vi "svc_ Octave Spectrum Labels and Units.vi"(9 "octave info":T1={"standard"=enum."ANSI S1.11", "bandwidth"=enum."1 octave", "low band"=0, "high band"=0, "weighting filter"=0, "dB reference"=0.0, "dB On"=FALSE, "unit label"="", "channel name"="", "description"="", "engineering units"=1, "custom label"="", "spectrum type"=enum."magnitude", "spectral density"=FALSE, "filters settled"=FALSE} {"engineering units" items=["custom..."=0, "V"=1, "A"=21, "C"=30, "pC"=31, "s"=32, "-"=29, "Pa"=2, "N"=20, "g"=3, "m/s^2"=4, "m/s"=5, "m"=6, "mm/s"=12, "mm"=13, "micron/s"=14, "micron"=15, "in/s^2"=7, "in/s"=8, "in"=9, "mil/s"=10, "mil"=11, "rad/s^2"=16, "rad/s"=17, "rad"=18, "deg/s^2"=26, "deg/s"=27, "deg"=28, "RPM"=22, "cycle/s^2"=23, "Hz"=24, "cycle"=25, "strain"=19]; "dB reference" format="%.2e"; "weighting filter" items=["Linear", "A-weighting", "B-weighting", "C-weighting", "ITU-R 468-4", "Dolby", "CCITT", "C-message", "Wb", "Wc", "Wd", "We", "Wf", "Wh", "Wj", "Wk", "Wm", "AES17 20 kHz lowpass", "AES17 40 kHz lowpass", "AES17 20 kHz highpass", "AES17 40 kHz highpass"]}) -> (1 "octave info out":T1={"standard"=enum."ANSI S1.11", "bandwidth"=enum."1 octave", "low band"=0, "high band"=0, "weighting filter"=0, "dB reference"=0.0, "dB On"=FALSE, "unit label"="", "channel name"="", "description"="", "engineering units"=1, "custom label"="", "spectrum type"=enum."magnitude", "spectral density"=FALSE, "filters settled"=FALSE} {"engineering units" items=["custom..."=0, "V"=1, "A"=21, "C"=30, "pC"=31, "s"=32, "-"=29, "Pa"=2, "N"=20, "g"=3, "m/s^2"=4, "m/s"=5, "m"=6, "mm/s"=12, "mm"=13, "micron/s"=14, "micron"=15, "in/s^2"=7, "in/s"=8, "in"=9, "mil/s"=10, "mil"=11, "rad/s^2"=16, "rad/s"=17, "rad"=18, "deg/s^2"=26, "deg/s"=27, "deg"=28, "RPM"=22, "cycle/s^2"=23, "Hz"=24, "cycle"=25, "strain"=19]; "dB reference" format="%.2e"; "weighting filter" items=["Linear", "A-weighting", "B-weighting", "C-weighting", "ITU-R 468-4", "Dolby", "CCITT", "C-message", "Wb", "Wc", "Wd", "We", "Wf", "Wh", "Wj", "Wk", "Wm", "AES17 20 kHz lowpass", "AES17 40 kHz lowpass", "AES17 20 kHz highpass", "AES17 40 kHz highpass"]}, 2 "unit label":string)   [LabVIEW 2017]
uses:
  <vilib>/addons/_NISVFA/_Shared subVIs/Controls/svc_Octave Info.ctl
  <vilib>/addons/_NISVFA/_Shared subVIs/Controls/svc_Octave Standard.ctl
  <vilib>/addons/_NISVFA/_Shared subVIs/Controls/svc_Weighting Filter Text Ring.ctl
  <vilib>/addons/_NISVFA/_Shared subVIs/Controls/svc_Engineering Units Text Ring.ctl
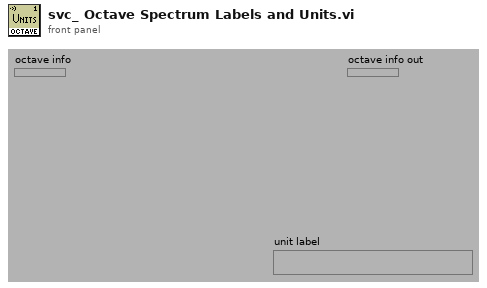
[diagram p1: front panel]
types:
  T1 = typedef "svc_Octave Info.ctl" = cluster{"standard":T2, "bandwidth":enum16{"1 octave", "1/3 octave", "1/6 octave", "1/12 octave", "1/24 octave"}, "low band":i32, "high band":i32, "weighting filter":T3, "dB reference":dbl, "dB On":bool, "unit label":string, "channel name":string, "description":string, "engineering units":T4, "custom label":string, "spectrum type":enum16{"power", "magnitude"}, "spectral density":bool, "filters settled":bool}
  T2 = typedef "svc_Octave Standard.ctl" = enum16{"ANSI S1.11", "IEC 61260"}
  T3 = typedef "svc_Weighting Filter Text Ring.ctl" = u16
  T4 = typedef "svc_Engineering Units Text Ring.ctl" = u16
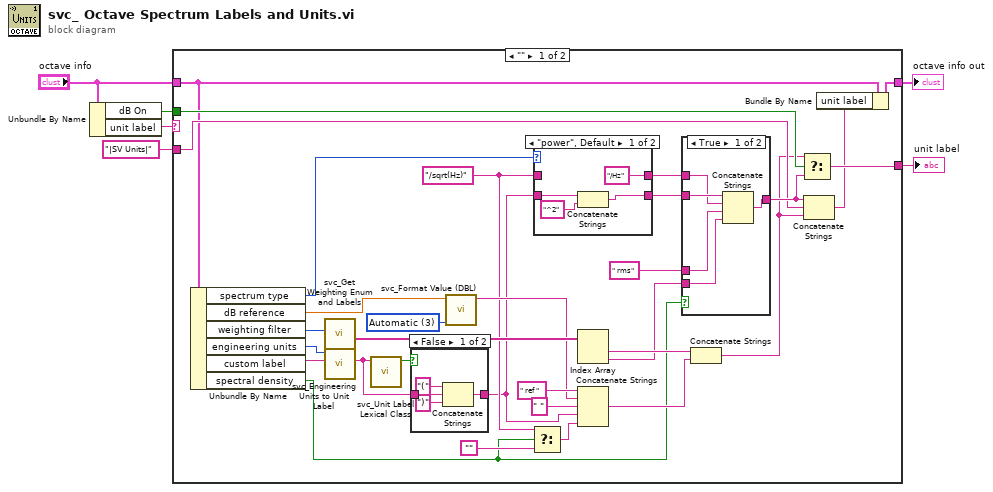
[diagram p0: block diagram]
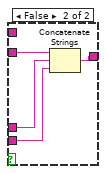
[diagram p3: hidden frame]
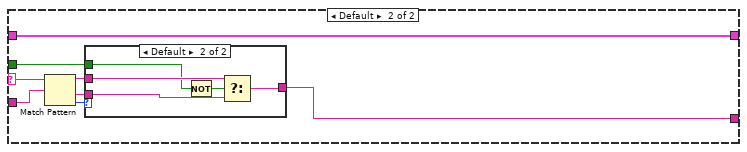
[diagram p5: hidden frame]
diagram:
  n1 = Unbundle By Name("octave info") -> ("dB On"=w2:bool, "unit label"=w4:string)
  n2 = case shown="\"\"" w4 {
    selector: w4 -> [_ w62]
    tunnel: [w34 w59] -> w6
    tunnel: "octave info" -> [w18 w59]
    tunnel: "|SV Units|" ("string") -> [w30 w61]
    tunnel: w2 -> [w33 w60]
    tunnel: [w32 w58] -> w1
    frame "" {
      w15 = "/sqrt(Hz)"
      w23 = i16 3 items=["Engineering", "Exponential", "Fractional", "Automatic"] ("number format")
      n3 = Unbundle By Name(w18) -> ("spectrum type"=w13:enum16{"power", "magnitude"}, "dB reference"=w12:dbl, "weighting filter"=w11:T3, "engineering units"=w10:T4, "custom label"=w9:string, "spectral density"=w7:bool)
      n4 = call <vilib>:"svc_Get Weighting Enum and Labels.vi"("weighting filter"=w11) -> ("weighting subarray"=w26:string[])  [unwired: 7 in, 1 out]
      n5 = call <vilib>:"svc_Engineering Units to Unit Label.vi"("custom label"=w9, "engineering units"=w10) -> ("unit label"=w17:string)  [unwired: 8 in, 1 out]
      n6 = call <vilib>:"svc_Unit Label Lexical Class.vi"("unit label"=w17) -> ("letters only?"=w16:bool)  [unwired: 6 in]
      n7 = case shown="False" w16 {
        tunnel: w17 -> [w41 w42]
        tunnel: [w40 w42] -> w8
        frame False {
          n8 = Concatenate Strings("(" ("string"), w41, ")" ("string")) -> (w40:string)
        }
        frame True {
        }
      }
      n9 = call <vilib>:"svc_Format Value (DBL).vi"("number format"=w23, "dB reference"=w12) -> ("format string"=w20:string)  [unwired: 9 in]
      n10 = Select(t=w15, s=w7, f="") -> (s? t:f=w14:string)
      n11 = case shown="\"power\", Default" w13 {
        tunnel: w8 -> [w53 w57]
        tunnel: [w54 w57] -> w37
        tunnel: ["/Hz" w56] -> w35
        tunnel: w15 -> [_ w56]
        frame "power", Default {
          n12 = Concatenate Strings(w53, "^2") -> (w54:string)
        }
        frame "magnitude" {
        }
      }
      n13 = Index Array(array=w26) -> (element #1=w25:string, element #2=w19:string)  [unwired: 2 in]
      n14 = Concatenate Strings(" ref ", w20, " " ("Substring"), w8, w14) -> (w24:string)
      n15 = case shown="True" w7 {
        tunnel: w37 -> [w47 w51]
        tunnel: [w46 w50] -> w31
        tunnel: w19 -> [w45 w49]
        tunnel: " rms" -> [w44 w48]
        tunnel: w35 -> [w43 _]
        frame True {
          n16 = Concatenate Strings(w47, w43, w44, w45) -> (w46:string)
        }
        frame False {
          n17 = Concatenate Strings(w51, w48, w49) -> (w50:string)
        }
      }
      n18 = Concatenate Strings(w25, w24) -> (w29:string)
      n19 = Select(t=w29, s=w33, f=w31) -> (s? t:f=w32:string)
      n20 = Concatenate Strings(w31, w30, w29) -> (w28:string)
      n21 = Bundle By Name(cluster=w18, "unit label"=w28) -> (w34:T1)
    }
    frame Default {
      n22 = Match Pattern(string=w62, regular expression=w61) -> (before substring=w65:string, after substring=w64:string, offset past match=w63:i32)  [unwired: 1 in, 1 out]
      n23 = case shown="Default" w63 {
        tunnel: w65 -> [w66 w71]
        tunnel: w64 -> [_ w70]
        tunnel: [w66 w69] -> w58
        tunnel: w60 -> [_ w68]
        frame -1 {
        }
        frame Default {
          n24 = Not(x=w68) -> (.not. x?=w67:bool)
          n25 = Select(t=w71, s=w67, f=w70) -> (s? t:f=w69:string)
        }
      }
    }
  }
  "octave info out" <- w6
  "unit label" <- w1
